vi "JYTurret.vi"(3 "error in (no error)":errorcluster, 4 "Grating Index":i32, 5 "JYMONOLib.IJYMonoReqd In":refnum<k7>) -> (0 "error out":errorcluster, 1 "Busy":bool, 2 "JYMONOLib.IJYMonoReqd Out":refnum<k7>)   [LabVIEW 2017]
doc: "JYTurret.vi\n\nMove the turret to select a new grating\n\nInputs -\nRefNum In - LabView automation RefNum \nUnique ID\nInput Error Cluster \n\n--------------------------------------------\nOutputs -\nRefNum Out -\nBusy Flag\nOutput Error Cluster"
panel:
  out "UseUniqueID":bool
  in  "UniqueID":string
  in  "Mode Select":bool caption="Input Select"
  # "Local / Front Panel Mode"
  # "Remote / Program Mode"
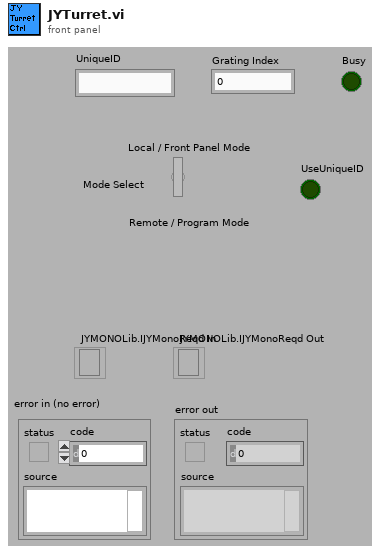
[diagram p1: front panel]
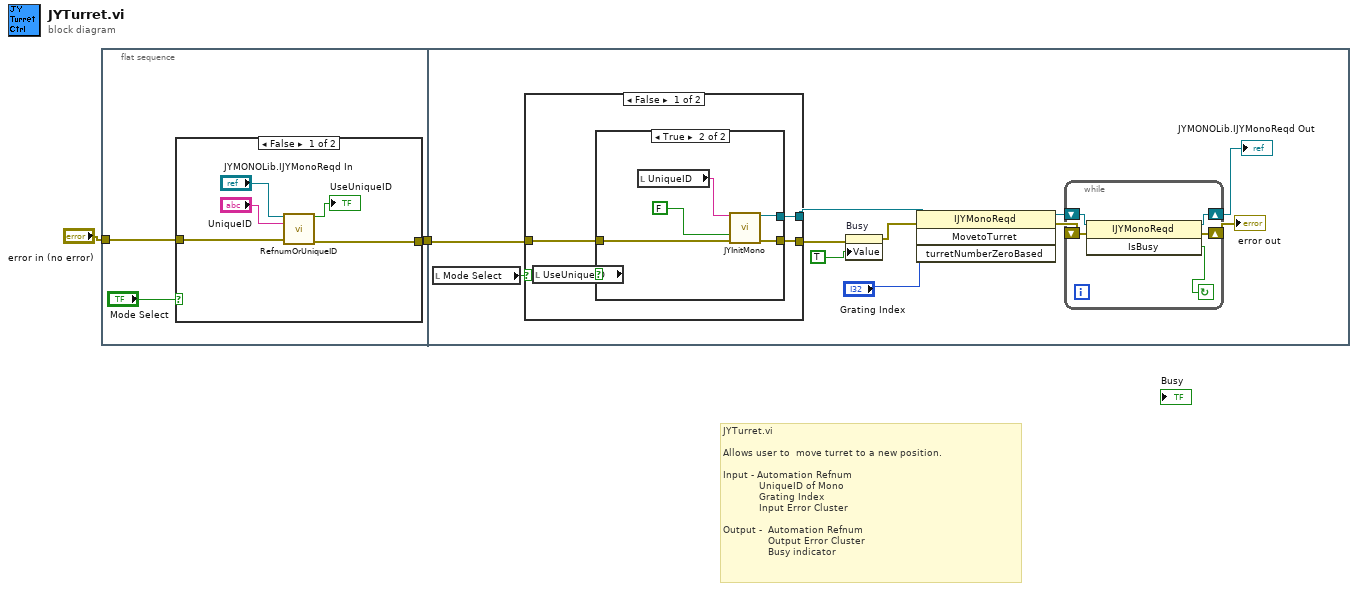
[diagram p0: block diagram]
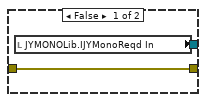
[diagram p3: hidden frame]
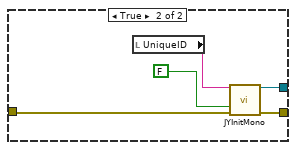
[diagram p4: hidden frame]
diagram:
  # "JYTurret.vi\n\nAllows user to  move turret to a new position.  \n\nInput - Automation Refnum \n            UniqueID of Mono\n            Grating Index\n            Input Error Cluster\n\nOutput -  Automation Refnum\n               Output Error Cluster\n               Busy indicator"
  n1 = flat-sequence {
    tunnel: "error in (no error)" -> [w4]
    tunnel: [w3] -> w1
    tunnel: w1 -> [w21]
    frame #0 {
      n2 = case shown="False" "Mode Select" {
        tunnel: w4 -> [w7 w11]
        tunnel: [w6 w11] -> w3
        frame False {
          n3 = call "RefnumOrUniqueID.vi"("Refnum IN"="JYMONOLib.IJYMonoReqd In", "String in"="UniqueID", "error in (no error)"=w7) -> ("UseUniqueID"=→"UseUniqueID":bool, "error out"=w6:errorcluster)  [unwired: 11 out]
        }
        frame True {
        }
      }
    }
    frame #1 {
      n4 = local read "Mode Select"() -> (w22:bool)
      n5 = case shown="False" w22 {
        tunnel: w21 -> [w30 w41]
        tunnel: [w29 w40] -> w19
        tunnel: [w28 w39] -> w20
        frame False {
          n6 = local read "UseUniqueID"() -> (w31:bool)
          n7 = case shown="True" w31 {
            tunnel: w30 -> [w33 w36]
            tunnel: [w33 w35] -> w29
            tunnel: [w32 w34] -> w28
            frame False {
              n8 = local read "JYMONOLib.IJYMonoReqd In"() -> (w32:refnum<k7>)
            }
            frame True {
              n9 = local read "UniqueID"() -> (w38:string)
              n10 = call "JYInitMono.vi"("Unique ID"=w38, "Force Init"=FALSE, "error in (no error)"=w36) -> ("Mono RefNum out"=w34:refnum<k7>, "error out"=w35:errorcluster)  [unwired: 1 in, 10 out]
            }
          }
        }
        frame True {
          n11 = local read "UniqueID"() -> (w43:string)
          n12 = call "JYInitMono.vi"("Unique ID"=w43, "Force Init"=FALSE, "error in (no error)"=w41) -> ("Mono RefNum out"=w39:refnum<k7>, "error out"=w40:errorcluster)  [unwired: 1 in, 10 out]
        }
      }
      n13 = property on="Busy" class="Bool (strict)"(error in=w19, "Value"=TRUE ("Busy")) -> (error out=w18:errorcluster)  [unwired: 1 in, 1 out]
      n14 = invoke class="IJYMonoReqd" method="MovetoTurret"(reference=w20, error in=w18, "turretNumberZeroBased"="Grating Index") -> (reference out=w13:refnum<k7>, error out=w16:errorcluster)  [unwired: 1 in, 2 out]
      n15 = while {
        shift-right: [w24] -> w15
        shift-left: w16 -> [w25]
        shift-right: [w26] -> w12
        shift-left: w13 -> [w27]
        stop <- w23 continue-if-true
        n16 = invoke class="IJYMonoReqd" method="IsBusy"(reference=w27, error in=w25) -> (reference out=w26:refnum<k7>, error out=w24:errorcluster, "IsBusy"=w23:bool)  [unwired: 1 in]
      }
      "JYMONOLib.IJYMonoReqd Out" <- w12
      "error out" <- w15
    }
  }
